vi "Input_Instrument_Positions.vi"(1 "Filepath to Save":path) -> ()   [LabVIEW 2022 SP3]
uses:
  Globals/Meas_global.vi
  Globals/Constants_global.vi
  Globals/Trav_pos_global.vi
  Controls/Initial Positions.ctl
  On_Axes_Cluster.ctl
  Controls/ok_button.ctl
panel:
  in  "On Axes":T1
  in  "OK":T2
  in  "Instrument positions when the traverse is at its origin":T3(array[cluster])=[{"Name"="", "X"=0.0, "Y"=0.0, "Z"=0.0, "Mounted On"=0, "On Axes"=enum."X Y Z"}] {"Mounted On" items=["Position N/A", "No Traverse", "A_Tunnel", "Aero_Enclosure", "Aero_Sting", "Aero_ThroughWall", "Aero_Tunnel", "Angle_Calibrator", "B_Tunnel", "D_Tunnel", "Dummy_Traverse", "EnFlo_Stack", "EnFlo_Tunnel", "EnFlo_Turntable", "Laser_Meas_Traverse", "Pitch_Yaw", "PIV_Traverse", "Tank"]; "Z" format="%#.2f"; "Y" format="%#.2f"; "X" format="%#.2f"}
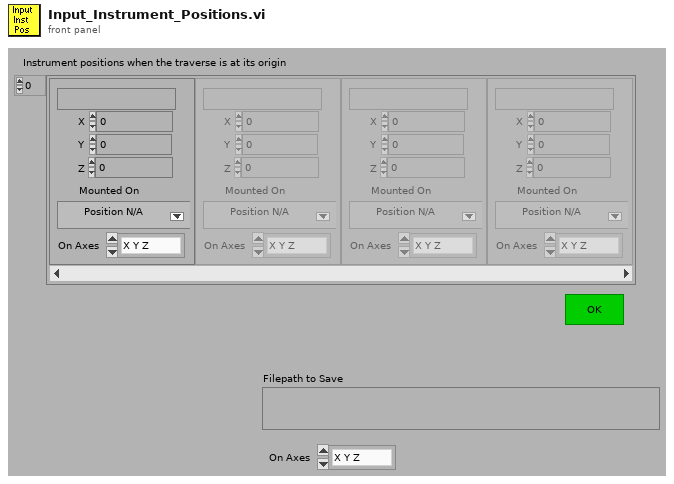
[diagram p1: front panel]
types:
  T1 = typedef "On_Axes_Cluster.ctl" = enum16{"X Y Z", "X Y", "X"}
  T2 = typedef "ok_button.ctl" = bool
  T3 = cluster{"Name":string, "X":dbl, "Y":dbl, "Z":dbl, "Mounted On":u16, "On Axes":T1}[]
  T4 = typedef "Analysis_info_cluster.ctl" = cluster{"Colour":u32, "Inst type":T5, "Inst name":string, "Symbol":string, "Code name":string, "Extra Info":string, "Inst Array":T6, "Extra Titles":string[], "Extra Values":string[], "U":dbl, "u^2":dbl, "u^3":dbl, "u^4":dbl, "Skew_u":dbl, "Kurt_u":dbl, "Sd Error in Mean":dbl, "% u'/U":dbl, "X":dbl, "Y":dbl, "Z":dbl, "Timescale integral Estimate":dbl, "Sd Error in Variance":dbl, "Calib File":path, "Calib Constants":dbl[], "Output Position":bool, "Stats":enum16{"None", "Basic", "Full"}, "Av Sampling Rate":dbl, "Av No of Samples":dbl, "Total Meas Time (s)":dbl, "ADAM Ch Name":string, "Max value":dbl, "Min value":dbl, "Req Sample Rate Hz":dbl, "Sync Delay Time (s)":dbl, "Ch No":i16, "Device":string, "Use Latest Calib":bool, "Port":string, "Metadata Ch Names":string[], "Metadata Ch Values":string[], "Label":string}
  T5 = typedef "Inst_type.ctl" = enum16{"Raw voltage", "Raw with zero offsetting", "Propeller anemometer", "Pressure Transducer", "Pitot-static tube", "Hot wire", "Cross wire 1", "Cross wire 2", "Generic Linear", "Generic Polynomial", "Generic BackPoly", "Fast FID", "Thermocouple", "Cold wire", "Pulsed Wire", "LDA Vel", "LDA Tran time", "LDA Arr time", "Microphone"}
  T6 = typedef "Instrument_Array.ctl" = enum16{"PWA", "LDA", "Analogue"}
  T7 = typedef "Initial Positions.ctl" = cluster{"Initial XYZ":sgl[], "Traverse Setup":string, "On Axes":string, "Identity String":string}
  T8 = cluster{"Name":string, "X":dbl, "Y":dbl, "Z":dbl, "Mounted On":u16, "On Axes":T1}
  T9 = cluster{"Values[0]":dbl, "Values[1]":dbl, "Values[2]":dbl}
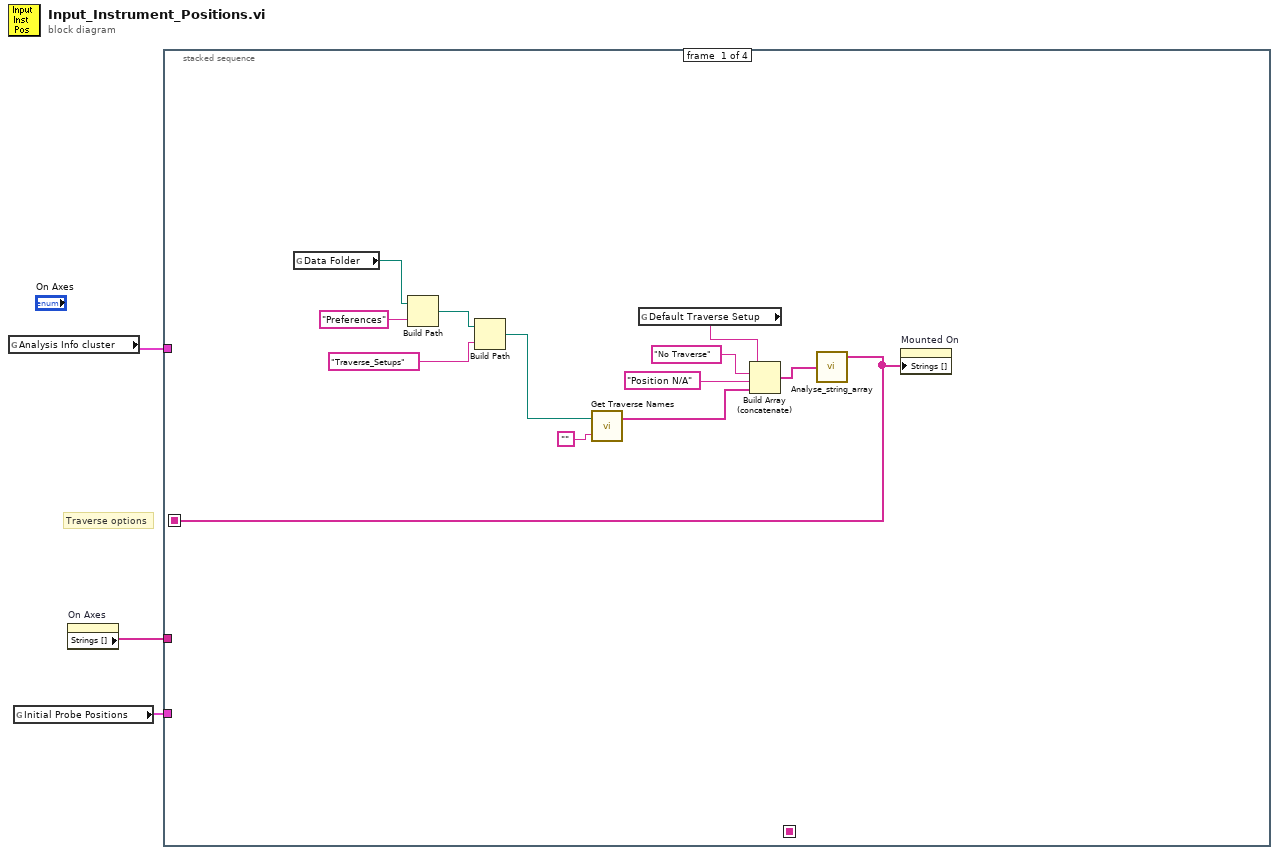
[diagram p0: block diagram]
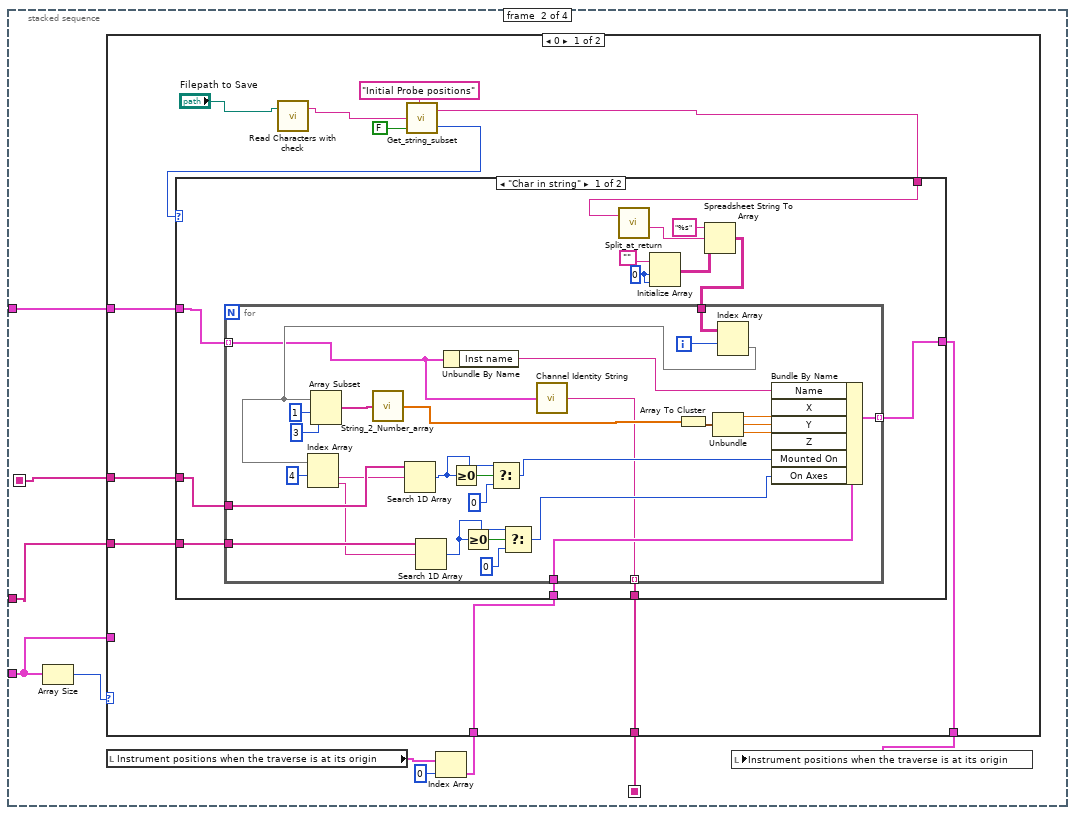
[diagram p2: hidden frame]
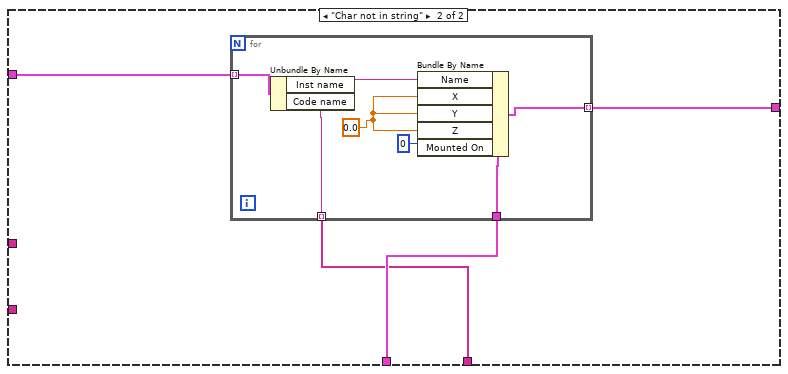
[diagram p3: hidden frame]
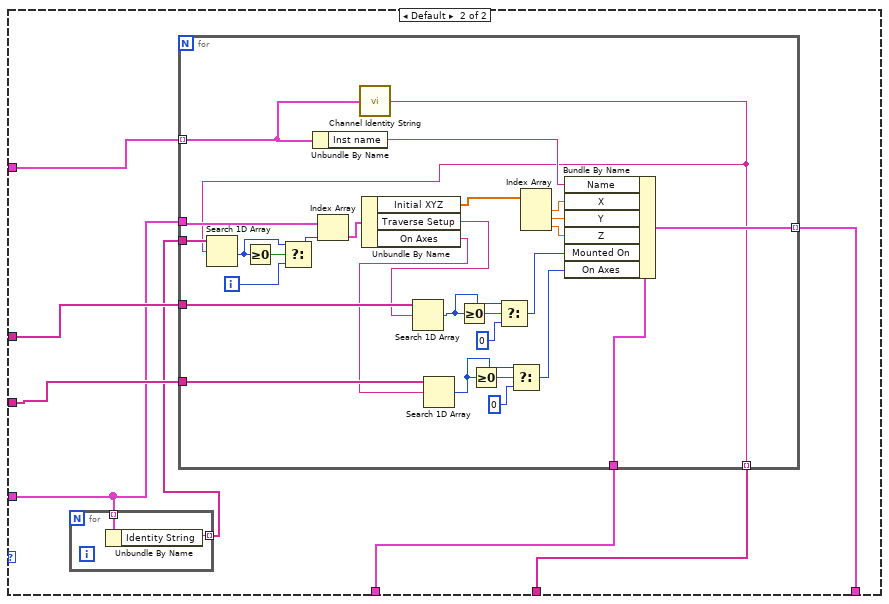
[diagram p4: hidden frame]
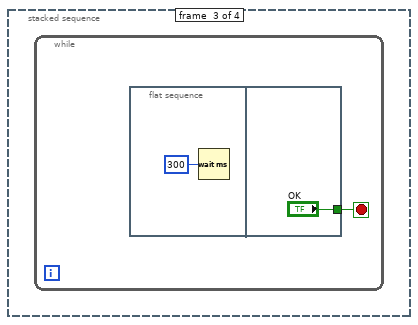
[diagram p5: hidden frame]
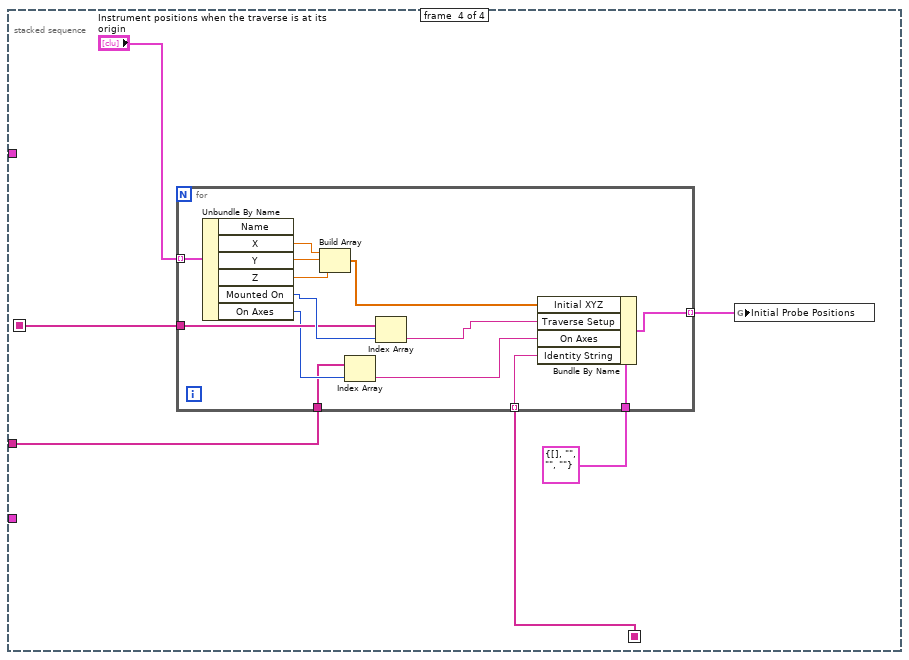
[diagram p6: hidden frame]
diagram:
  # "Traverse options"
  n1 = global read "Meas_global.vi" "Analysis Info cluster"() -> (w3:T4[])
  n2 = global read "Meas_global.vi" "Initial Probe Positions"() -> (w1:T7[])
  n3 = property on="On Axes" class="Enum (strict)"() -> ("Strings []"=w2:string[])  [unwired: 2 in, 2 out]
  n4 = stacked-sequence {
    seq-local: [w8 _ _ _] -> [_ w24 _ w136]
    seq-local: [_ w16 _ _] -> [_ _ _ w132]
    tunnel: w3 -> [_ w25 _ _]
    tunnel: w2 -> [_ w23 _ w135]
    tunnel: w1 -> [_ w20 _ _]
    frame #0 {
      n5 = global read "Constants_global.vi" "Data Folder"() -> (w12:path)
      n6 = Build Path(base path=w12, name or relative path="Preferences") -> (appended path=w14:path)
      n7 = Build Path(base path=w14, name or relative path="Traverse_Setups") -> (appended path=w6:path)
      n8 = call "Get Traverse Names.vi"("Traverse name"="", "Traverse\nSetup\nFolder"=w6) -> ("Traverse Names"=w5:string[])  [unwired: 1 out]
      n9 = global read "Trav_pos_global.vi" "Default Traverse Setup"() -> (w11:string)
      n10 = Build Array (concatenate)(w11, "No Traverse" ("element"), "Position N/A" ("element"), w5) -> (w9:string[])
      n11 = call "Analyse_string_array.vi"("String array"=w9) -> ("Unique strings"=w8:string[])  [unwired: 2 out]
      n12 = property on="Mounted On" class="Ring (strict)"("Strings []"=w8) -> ()  [unwired: 2 in, 2 out]
    }
    frame #1 {
      n13 = Array Size(array=w20) -> (size(s)=w22:i32)
      n14 = local read "Instrument positions when the traverse is at its origin"() -> (w19:T3)
      n15 = Index Array(array=w19, index=0) -> (element=w17:T8)
      n16 = case shown="0" w22 {
        tunnel: w25 -> [w37 w97]
        tunnel: w24 -> [w36 w96]
        tunnel: w23 -> [w31 w95]
        tunnel: [w30 w94] -> w21
        tunnel: w20 -> [_ w93]
        tunnel: w17 -> [w29 w98]
        tunnel: [w28 w91] -> w16
        frame 0 {
          n17 = call "Read Characters with check.vi"("file (use dialog)"="Filepath to Save") -> ("Read String"=w26:string)  [unwired: 1 in, 1 out]
          n18 = call "Get_string_subset.vi"("Show Dialog?"=FALSE, "String to split"=w26, "File Label"="Initial Probe positions") -> ("Status"=w32:enum16{"Char in string", "Char not in string"}, "Output string"=w33:string)  [unwired: 1 in]
          n19 = case shown="\"Char in string\"" w32 {
            tunnel: w37 -> [w41 w83]
            tunnel: w29 -> [w45 w82]
            tunnel: [w44 w81] -> w30
            tunnel: w36 -> [w43 _]
            tunnel: w33 -> [w42 _]
            tunnel: w31 -> [w39 _]
            tunnel: [w38 w80] -> w28
            frame "Char in string" {
              w47 = 0 ("Dimension Size")
              n20 = call "Split_at_return.vi"("String"=w42) -> ("after substring"=w50:string)  [unwired: 1 in, 3 out]
              n21 = Initialize Array("", w47, w47) -> (w46:string[][])
              n22 = Spreadsheet String To Array(format string="%s", spreadsheet string=w50, array type (2D Dbl)=w46) -> (array=w40:string[][])  [unwired: 1 out]
              n23 = for {
                tunnel: [w70] -> w44 mode=indexing
                tunnel: w45 -> [w69]
                tunnel: w43 -> [w68]
                tunnel: w41 -> [w52] mode=indexing
                tunnel: w40 -> [w61]
                tunnel: w39 -> [w58]
                tunnel: [w51] -> w38 mode=indexing
                i -> [w60]
                n24 = Unbundle By Name(w52) -> ("Inst name"=w62:string)
                n25 = call "Channel Identity String.vi"("Analysis Cluster"=w52) -> ("Identity String"=w51:string)
                n26 = Index Array(array=w61, index (row)=w60) -> (element=w59:string[])  [unwired: 1 in]
                n27 = Index Array(array=w59, index #1=4 ("index")) -> (element #1=w67:string, element #2=w57:string)  [unwired: 1 in]
                n28 = Array Subset(array=w59, index=1, length=3) -> (w77:string[])
                n29 = call "String_2_Number_array.vi"("Input String"=w77) -> ("Values"=w76:dbl[])
                n30 = Search 1D Array(1D array=w68, element=w67) -> (index of element=w65:i32)  [unwired: 1 out]
                n31 = Search 1D Array(1D array=w58, element=w57) -> (index of element=w54:i32)  [unwired: 1 out]
                n32 = Greater Or Equal To 0?(x=w65) -> (x >= 0?=w66:bool)
                n33 = Greater Or Equal To 0?(x=w54) -> (x >= 0?=w55:bool)
                n34 = Select(t=w65, s=w66, f=0) -> (s? t:f=w63:i32)
                n35 = Select(t=w54, s=w55, f=0) -> (s? t:f=w53:i32)
                n36 = Array To Cluster(array=w76) -> (cluster=w75:T9)
                n37 = Unbundle(w75) -> ("Values[0]"=w74:dbl, "Values[1]"=w73:dbl, "Values[2]"=w72:dbl)
                n38 = Bundle By Name(cluster=w69, "Name"=w62, "X"=w74, "Y"=w73, "Z"=w72, "Mounted On"=w63, "On Axes"=w53) -> (w70:T8)
              }
            }
            frame "Char not in string" {
              n39 = for {
                tunnel: w83 -> [w87] mode=indexing
                tunnel: w82 -> [w86]
                tunnel: [w85] -> w81 mode=indexing
                tunnel: [w84] -> w80 mode=indexing
                w88 = 0.0 ("Z")
                n40 = Unbundle By Name(w87) -> ("Inst name"=w90:string, "Code name"=w84:string)
                n41 = Bundle By Name(cluster=w86, "Name"=w90, "X"=w88, "Y"=w88, "Z"=w88, "Mounted On"=u16 0) -> (w85:T8)
              }
            }
          }
        }
        frame Default {
          n42 = for {
            tunnel: w93 -> [w100] mode=indexing
            tunnel: [w99] -> w92 mode=indexing
            n43 = Unbundle By Name(w100) -> ("Identity String"=w99:string)
          }
          n44 = for {
            tunnel: w93 -> [w109]
            tunnel: w98 -> [w128]
            tunnel: w97 -> [w106] mode=indexing
            tunnel: w96 -> [w116]
            tunnel: w95 -> [w115]
            tunnel: [w110] -> w94 mode=indexing
            tunnel: w92 -> [w107]
            tunnel: [w105] -> w91 mode=indexing
            i -> [w102]
            n45 = Unbundle By Name(w106) -> ("Inst name"=w127:string)
            n46 = call "Channel Identity String.vi"("Analysis Cluster"=w106) -> ("Identity String"=w105:string)
            n47 = Search 1D Array(1D array=w107, element=w105) -> (index of element=w103:i32)  [unwired: 1 out]
            n48 = Greater Or Equal To 0?(x=w103) -> (x >= 0?=w104:bool)
            n49 = Select(t=w103, s=w104, f=w102) -> (s? t:f=w101:i32)
            n50 = Index Array(array=w109, index=w101) -> (element=w108:T7)
            n51 = Unbundle By Name(w108) -> ("Initial XYZ"=w126:sgl[], "Traverse Setup"=w114:string, "On Axes"=w113:string)
            n52 = Search 1D Array(1D array=w116, element=w114) -> (index of element=w121:i32)  [unwired: 1 out]
            n53 = Search 1D Array(1D array=w115, element=w113) -> (index of element=w117:i32)  [unwired: 1 out]
            n54 = Greater Or Equal To 0?(x=w121) -> (x >= 0?=w122:bool)
            n55 = Greater Or Equal To 0?(x=w117) -> (x >= 0?=w118:bool)
            n56 = Select(t=w121, s=w122, f=0) -> (s? t:f=w111:i32)
            n57 = Select(t=w117, s=w118, f=0) -> (s? t:f=w112:i32)
            n58 = Index Array(array=w126) -> (element #1=w125:sgl, element #2=w124:sgl, element #3=w123:sgl)  [unwired: 3 in]
            n59 = Bundle By Name(cluster=w128, "Name"=w127, "X"=w125, "Y"=w124, "Z"=w123, "Mounted On"=w111, "On Axes"=w112) -> (w110:T8)
          }
        }
      }
      n60 = local write "Instrument positions when the traverse is at its origin"(w21) -> ()
    }
    frame #2 {
      n61 = while {
        stop <- w129 stop-if-true
        n62 = flat-sequence {
          tunnel: ["OK"] -> w129
          frame #0 {
            n63 = Wait (ms)(milliseconds to wait=u32 300) -> ()  [unwired: 1 out]
          }
          frame #1 {
          }
        }
      }
    }
    frame #3 {
      n64 = for {
        tunnel: "Instrument positions when the traverse is at its origin" -> [w151] mode=indexing
        tunnel: w136 -> [w146]
        tunnel: w135 -> [w144]
        tunnel: T7 {"Initial XYZ"=[], "Traverse Setup"="", "On Axes"="", "Identity String"=""} ("Initial Positions") -> [w143]
        tunnel: [w139] -> w133 mode=indexing
        tunnel: w132 -> [w138] mode=indexing
        n65 = Unbundle By Name(w151) -> ("X"=w150:dbl, "Y"=w149:dbl, "Z"=w148:dbl, "Mounted On"=w147:u16, "On Axes"=w145:T1)  [unwired: 1 out]
        n66 = Build Array(w150, w149, w148) -> (w142:dbl[])
        n67 = Index Array(array=w144, index=w145) -> (element=w140:string)
        n68 = Index Array(array=w146, index=w147) -> (element=w141:string)
        n69 = Bundle By Name(cluster=w143, "Initial XYZ"=w142, "Traverse Setup"=w141, "On Axes"=w140, "Identity String"=w138) -> (w139:T7)
      }
      n70 = global write "Meas_global.vi" "Initial Probe Positions"(w133) -> ()
    }
  }
